vi "Read Routines.vi"(8 "error in (no error)":errorcluster, 11 "Assembly Run in":refnum<class "Assembly Run.lvclass">) -> (0 "error out":errorcluster, 2 "Routines":refnum<class "Routine.lvclass">[](array[class]), 3 "Assembly Run out":refnum<class "Assembly Run.lvclass">)   [LabVIEW 2016, in "Assembly Run.lvclass"]
uses:
  Assembly Run.lvclass
  Routine/Routine.lvclass
  Assembly Run.lvclass/Assembly Run.ctl
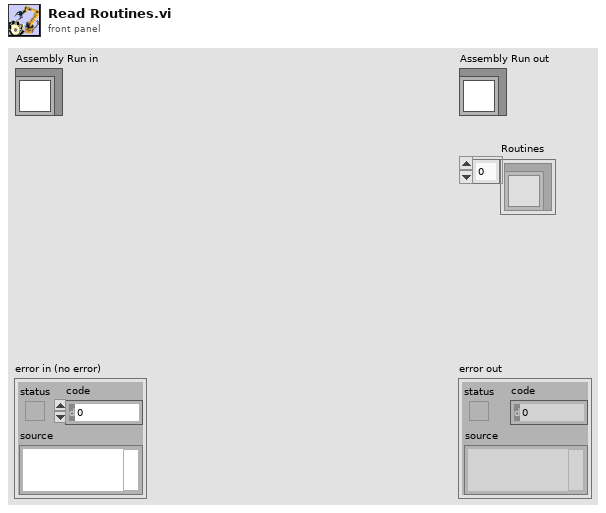
[diagram p1: front panel]
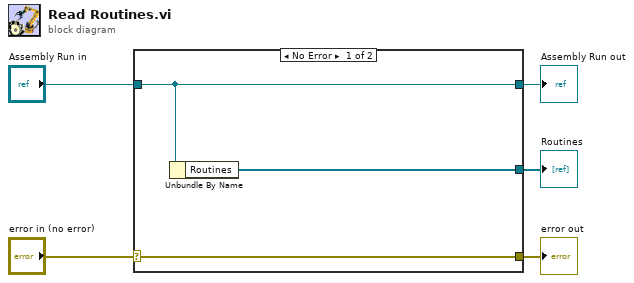
[diagram p0: block diagram]
diagram:
  n1 = case shown="No Error" "error in (no error)" {
    selector: "error in (no error)" -> [w8 w9]
    tunnel: [w8 w9] -> w4
    tunnel: [w7 w10] -> w2
    tunnel: "Assembly Run in" -> [w7 w10]
    tunnel: [w6 _] -> w1
    frame No Error {
      n2 = Unbundle By Name(w7) -> ("Routines"=w6:refnum<class "Routine.lvclass">[])
    }
    frame Error {
    }
  }
  "error out" <- w4
  "Assembly Run out" <- w2
  "Routines" <- w1
